vi "classify plclass.vi"(8 "error in":errorcluster, 10 "class cache data in":T1, 11 "Class Ancestry":path[](array[path])) -> (0 "error out":errorcluster, 2 "class cache data out":T1)   [LabVIEW 2013, in "PL_class cache.lvlib"]
uses:
  PL_class cache.lvlib
  cached class information.ctl
  target class metadata.ctl
  class metadata.ctl
  <vilib>/NI/Tag Bus Module Framework/root configuration/Target Types.ctl
  Configuration Editor/Classes/Targets/Targets.lvclass
  <vilib>/NI/Configuration Framework/serializable configuration/NISE_CEF_serializable configuration.lvclass
  Configuration Editor/Classes/Engine Parent/Engine Parent Editor Node.lvclass
  <vilib>/NI/Tag Bus Module Framework/root configuration/TBM configuration.lvclass
  Configuration Editor/Classes/Module editor node/module editor node.lvclass
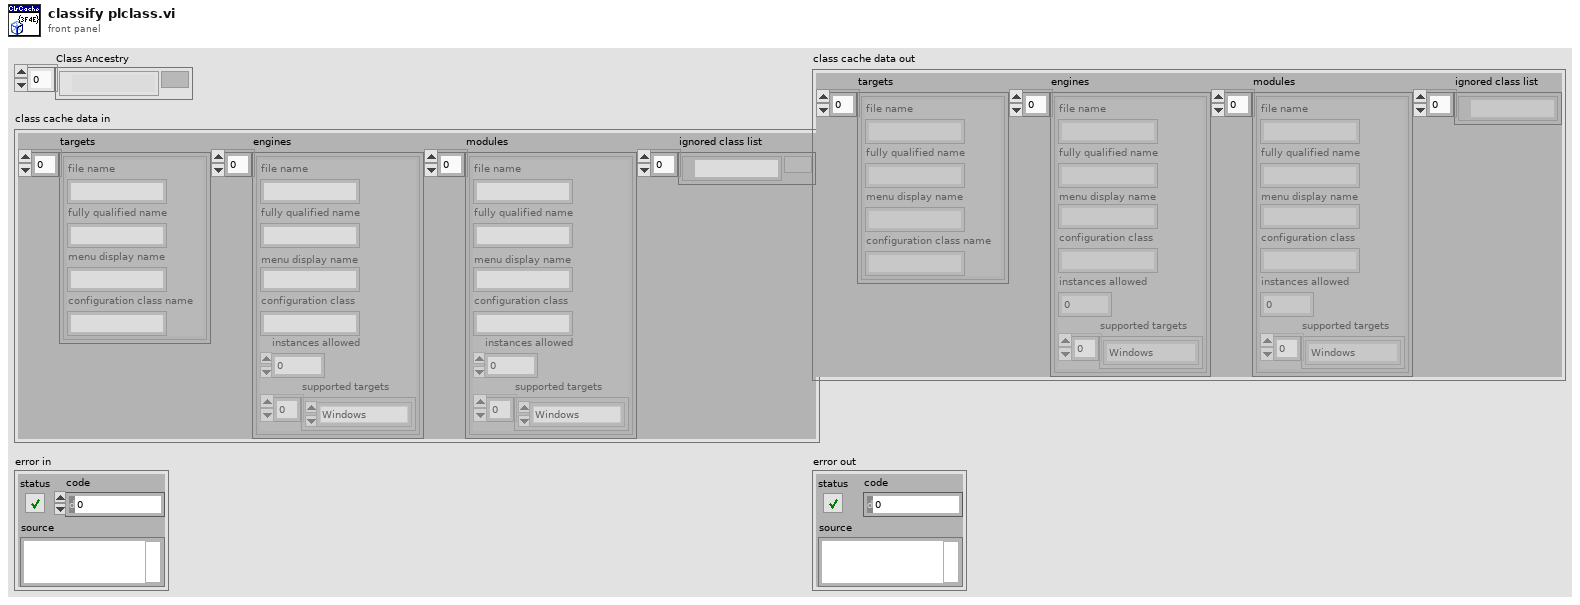
[diagram p1: front panel]
types:
  T1 = typedef "PL_class cache.lvlib/cached class information.ctl" = cluster{"targets":T2[], "engines":T3[], "modules":T3[], "ignored class list":path[]}
  T2 = typedef "PL_class cache.lvlib/target class metadata.ctl" = cluster{"file name":string, "fully qualified name":string, "menu display name":string, "configuration class name":string}
  T3 = typedef "PL_class cache.lvlib/class metadata.ctl" = cluster{"file name":string, "fully qualified name":string, "menu display name":string, "configuration class":string, "instances allowed":i32, "supported targets":T4[]}
  T4 = typedef "TBM configuration.lvclass/Target Types.ctl" = enum16{"Windows", "Mac", "Linux", "Linux RT ARM", "VxWorks", "Pharlap", "Other", "Linux RT x64"}
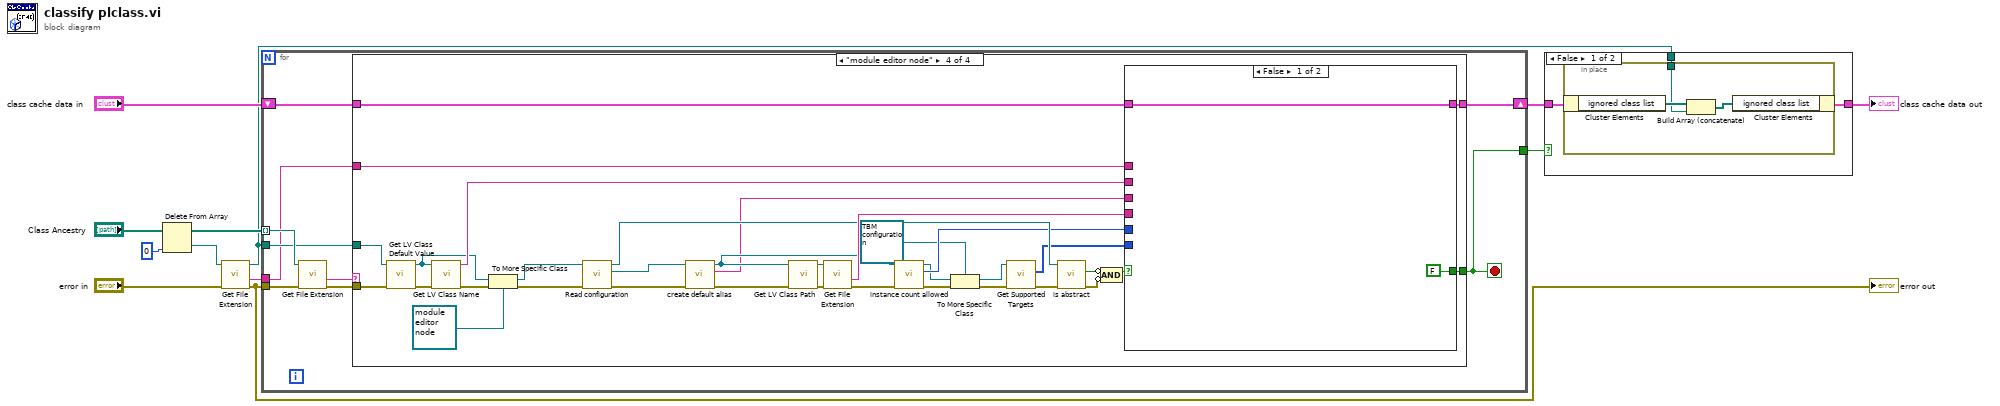
[diagram p0: block diagram]
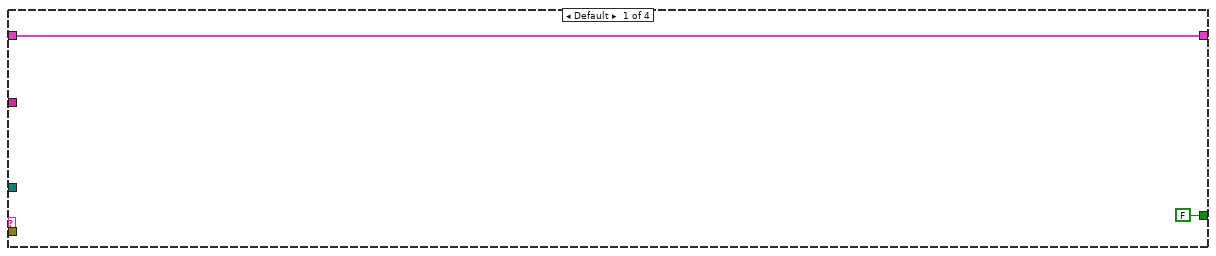
[diagram p3: hidden frame]
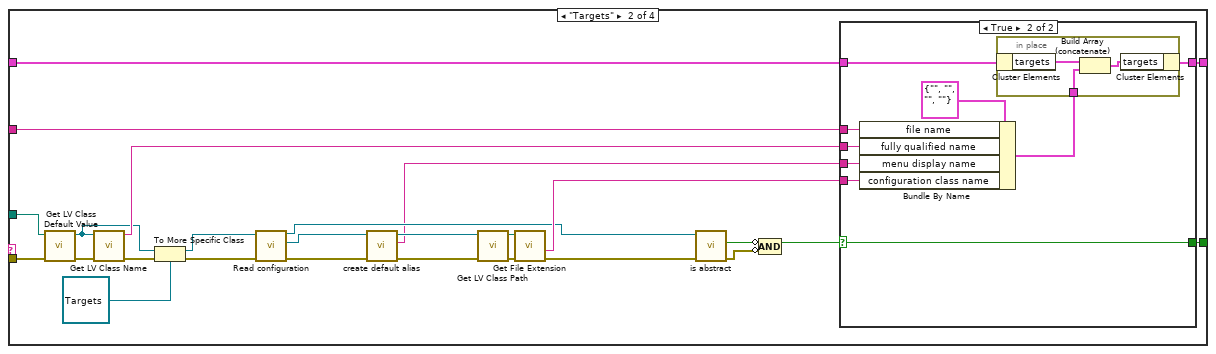
[diagram p4: hidden frame]
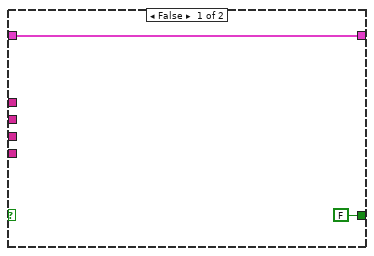
[diagram p5: hidden frame]
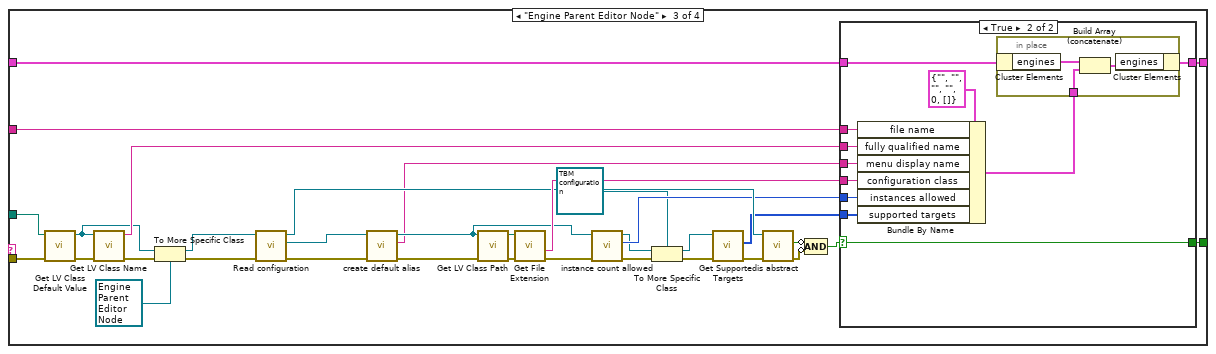
[diagram p6: hidden frame]
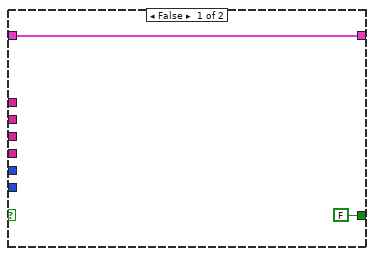
[diagram p7: hidden frame]
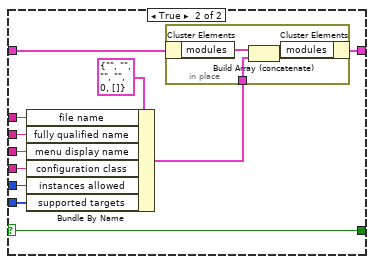
[diagram p8: hidden frame]
diagram:
  n1 = Delete From Array(array="Class Ancestry", index=0) -> (deleted portion=w4:path, array with subset deleted=w11:path[])  [unwired: 1 in]
  n2 = call <vilib>:"Get File Extension.vi"("error in (no error)"="error in", "file"=w4) -> ("error out"=w1:errorcluster, "filename without extension"=w2:string, "dup file"=w3:path)  [unwired: 6 in, 1 out]
  "error out" <- w1
  n3 = for {
    tunnel: w11 -> [w18] mode=indexing
    tunnel: w3 -> [w16]
    shift-right: [w20] -> w6
    shift-left: "class cache data in" -> [w21]
    tunnel: [w14] -> w7
    tunnel: w2 -> [w13]
    tunnel: w1 -> [w15]
    stop <- w14 stop-if-true
    n4 = call <vilib>:"Get File Extension.vi"("error in (no error)"=w15, "file"=w18) -> ("error out"=w19:errorcluster, "filename without extension"=w17:string)  [unwired: 6 in, 2 out]
    n5 = case shown="\"module editor node\"" w17 {
      tunnel: w21 -> [w23 w44 w93 w143]
      tunnel: [w23 w45 w94 w144] -> w20
      tunnel: w19 -> [_ w48 w96 w146]
      tunnel: [FALSE w49 w97 w147] -> w14
      tunnel: w16 -> [_ w47 w95 w145]
      tunnel: w13 -> [_ w43 w92 w142]
      frame Default {
      }
      frame "Targets" {
        n6 = call <vilib>:"Get LV Class Default Value.vi"("error in (no error)"=w48, "class path"=w47) -> ("error out"=w42:errorcluster, "object"=w39:refnum<class>)  [unwired: 8 in]
        n7 = call <vilib>:"Get LV Class Name.vi"("error in (no error)"=w42, "object"=w39) -> ("error out"=w40:errorcluster, "class name"=w41:string)  [unwired: 8 in]
        n8 = To More Specific Class(target class=refnum<class "Targets.lvclass"> refnum ("Targets"), reference=w39, error in=w40) -> (specific class reference=w24:refnum<class "Targets.lvclass">, error out=w25:errorcluster)
        n9 = call-dynamic "Read configuration.vi"("error in"=w25, "NISE_CEF_serializable node in"=w24) -> ("error out"=w37:errorcluster, "configuration"=w28:refnum<class "NISE_CEF_serializable configuration.lvclass">, "NISE_CEF_serializable node out"=w34:refnum<class "Targets.lvclass">)  [unwired: 7 in]
        n10 = call-dynamic "create default alias.vi"("error in"=w37, "configuration in"=w28) -> ("error out"=w29:errorcluster, "default alias"=w26:string, "configuration out"=w27:refnum<class "NISE_CEF_serializable configuration.lvclass">)  [unwired: 7 in]
        n11 = call <vilib>:"Get LV Class Path.vi"("error in (no error)"=w29, "object"=w27) -> ("error out"=w36:errorcluster, "class path"=w38:path)  [unwired: 8 in]
        n12 = call <vilib>:"Get File Extension.vi"("error in (no error)"=w36, "file"=w38) -> ("error out"=w33:errorcluster, "filename without extension"=w35:string)  [unwired: 6 in, 2 out]
        n13 = call-dynamic "is abstract.vi"("error in"=w33, "Targets in"=w34) -> ("error out"=w30:errorcluster, "abstract"=w32:bool)  [unwired: 7 in, 1 out]
        n14 = Compound Arithmetic op=AND(invert w32, invert w30) -> (w31:bool)
        n15 = case shown="True" w31 {
          selector: w31 -> [_ w52]
          tunnel: [FALSE w52] -> w49
          tunnel: [w51 w60] -> w45
          tunnel: w44 -> [w51 w59]
          tunnel: w43 -> [_ w57]
          tunnel: w41 -> [_ w56]
          tunnel: w26 -> [_ w54]
          tunnel: w35 -> [_ w53]
          frame False {
          }
          frame True {
            n16 = Bundle By Name(cluster=T2 {"file name"="", "fully qualified name"="", "menu display name"="", "configuration class name"=""} ("class metadata"), "file name"=w57, "fully qualified name"=w56, "menu display name"=w54, "configuration class name"=w53) -> (w55:T2)
            n17 = in-place {
              in-place-border: w55 -> [w61]
              n18 = in-place-cluster #1(w59) -> ("targets"=w63:T2[])
              n19 = Build Array (concatenate)(w63, w61) -> (w62:T2[])
              n20 = in-place-cluster #1("targets"=w62) -> (w60:T1)
            }
          }
        }
      }
      frame "Engine Parent Editor Node" {
        n21 = call <vilib>:"Get LV Class Default Value.vi"("error in (no error)"=w96, "class path"=w95) -> ("error out"=w91:errorcluster, "object"=w88:refnum<class>)  [unwired: 8 in]
        n22 = call <vilib>:"Get LV Class Name.vi"("error in (no error)"=w91, "object"=w88) -> ("error out"=w89:errorcluster, "class name"=w90:string)  [unwired: 8 in]
        n23 = To More Specific Class(target class=refnum<class "Engine Parent Editor Node.lvclass"> refnum ("Engine Parent.lvclass"), reference=w88, error in=w89) -> (specific class reference=w64:refnum<class "Engine Parent Editor Node.lvclass">, error out=w65:errorcluster)
        n24 = call-dynamic "Read configuration.vi"("error in"=w65, "NISE_CEF_serializable node in"=w64) -> ("error out"=w86:errorcluster, "configuration"=w68:refnum<class "NISE_CEF_serializable configuration.lvclass">, "NISE_CEF_serializable node out"=w83:refnum<class "Engine Parent Editor Node.lvclass">)  [unwired: 7 in]
        n25 = call-dynamic "create default alias.vi"("error in"=w86, "configuration in"=w68) -> ("error out"=w69:errorcluster, "default alias"=w66:string, "configuration out"=w67:refnum<class "NISE_CEF_serializable configuration.lvclass">)  [unwired: 7 in]
        n26 = call <vilib>:"Get LV Class Path.vi"("error in (no error)"=w69, "object"=w67) -> ("error out"=w85:errorcluster, "class path"=w87:path)  [unwired: 8 in]
        n27 = call <vilib>:"Get File Extension.vi"("error in (no error)"=w85, "file"=w87) -> ("error out"=w82:errorcluster, "filename without extension"=w84:string)  [unwired: 6 in, 2 out]
        n28 = call-dynamic "instance count allowed.vi"("error in"=w82, "configuration in"=w67) -> ("error out"=w79:errorcluster, "instances allowed"=w76:i32, "configuration out"=w71:refnum<class "NISE_CEF_serializable configuration.lvclass">)  [unwired: 7 in]
        n29 = To More Specific Class(target class=refnum<class "TBM configuration.lvclass"> refnum ("configuration in"), reference=w71, error in=w79) -> (specific class reference=w70:refnum<class "TBM configuration.lvclass">, error out=w73:errorcluster)
        n30 = call-dynamic "Get Supported Targets.vi"("error in"=w73, "configuration in"=w70) -> ("error out"=w78:errorcluster, "supported targets"=w77:T4[])  [unwired: 7 in, 1 out]
        n31 = call-dynamic "is abstract.vi"("error in"=w78, "Engine Parent Editor Node in"=w83) -> ("error out"=w74:errorcluster, "abstract"=w81:bool)  [unwired: 7 in, 1 out]
        n32 = Compound Arithmetic op=AND(invert w81, invert w74) -> (w75:bool)
        n33 = case shown="True" w75 {
          selector: w75 -> [_ w103]
          tunnel: [FALSE w103] -> w97
          tunnel: [w99 w110] -> w94
          tunnel: w93 -> [w99 w109]
          tunnel: w92 -> [_ w108]
          tunnel: w90 -> [_ w107]
          tunnel: w66 -> [_ w105]
          tunnel: w84 -> [_ w104]
          tunnel: w77 -> [_ w101]
          tunnel: w76 -> [_ w100]
          frame False {
          }
          frame True {
            n34 = Bundle By Name(cluster=T3 {"file name"="", "fully qualified name"="", "menu display name"="", "configuration class"="", "instances allowed"=0, "supported targets"=[]} ("class metadata"), "file name"=w108, "fully qualified name"=w107, "menu display name"=w105, "configuration class"=w104, "instances allowed"=w100, "supported targets"=w101) -> (w106:T3)
            n35 = in-place {
              in-place-border: w106 -> [w111]
              n36 = in-place-cluster #2(w109) -> ("engines"=w113:T3[])
              n37 = Build Array (concatenate)(w113, w111) -> (w112:T3[])
              n38 = in-place-cluster #2("engines"=w112) -> (w110:T1)
            }
          }
        }
      }
      frame "module editor node" {
        n39 = call <vilib>:"Get LV Class Default Value.vi"("error in (no error)"=w146, "class path"=w145) -> ("error out"=w141:errorcluster, "object"=w138:refnum<class>)  [unwired: 8 in]
        n40 = call <vilib>:"Get LV Class Name.vi"("error in (no error)"=w141, "object"=w138) -> ("error out"=w139:errorcluster, "class name"=w140:string)  [unwired: 8 in]
        n41 = To More Specific Class(target class=refnum<class "module editor node.lvclass"> refnum ("Component Parent.lvclass"), reference=w138, error in=w139) -> (specific class reference=w114:refnum<class "module editor node.lvclass">, error out=w115:errorcluster)
        n42 = call-dynamic "Read configuration.vi"("error in"=w115, "NISE_CEF_serializable node in"=w114) -> ("error out"=w136:errorcluster, "configuration"=w118:refnum<class "NISE_CEF_serializable configuration.lvclass">, "NISE_CEF_serializable node out"=w133:refnum<class "module editor node.lvclass">)  [unwired: 7 in]
        n43 = call-dynamic "create default alias.vi"("error in"=w136, "configuration in"=w118) -> ("error out"=w119:errorcluster, "default alias"=w116:string, "configuration out"=w117:refnum<class "NISE_CEF_serializable configuration.lvclass">)  [unwired: 7 in]
        n44 = call <vilib>:"Get LV Class Path.vi"("error in (no error)"=w119, "object"=w117) -> ("error out"=w135:errorcluster, "class path"=w137:path)  [unwired: 8 in]
        n45 = call <vilib>:"Get File Extension.vi"("error in (no error)"=w135, "file"=w137) -> ("error out"=w132:errorcluster, "filename without extension"=w134:string)  [unwired: 6 in, 2 out]
        n46 = call-dynamic "instance count allowed.vi"("error in"=w132, "configuration in"=w117) -> ("error out"=w130:errorcluster, "instances allowed"=w127:i32, "configuration out"=w122:refnum<class "NISE_CEF_serializable configuration.lvclass">)  [unwired: 7 in]
        n47 = To More Specific Class(target class=refnum<class "TBM configuration.lvclass"> refnum ("configuration in"), reference=w122, error in=w130) -> (specific class reference=w120:refnum<class "TBM configuration.lvclass">, error out=w123:errorcluster)
        n48 = call-dynamic "Get Supported Targets.vi"("error in"=w123, "configuration in"=w120) -> ("error out"=w129:errorcluster, "supported targets"=w128:T4[])  [unwired: 7 in, 1 out]
        n49 = call-dynamic "is abstract.vi"("error in"=w129, "module editor node in"=w133) -> ("error out"=w124:errorcluster, "abstract"=w131:bool)  [unwired: 7 in, 1 out]
        n50 = Compound Arithmetic op=AND(invert w131, invert w124) -> (w125:bool)
        n51 = case shown="False" w125 {
          selector: w125 -> [_ w153]
          tunnel: [FALSE w153] -> w147
          tunnel: [w149 w160] -> w144
          tunnel: w143 -> [w149 w159]
          tunnel: w142 -> [_ w158]
          tunnel: w140 -> [_ w157]
          tunnel: w116 -> [_ w155]
          tunnel: w134 -> [_ w154]
          tunnel: w128 -> [_ w151]
          tunnel: w127 -> [_ w150]
          frame False {
          }
          frame True {
            n52 = Bundle By Name(cluster=T3 {"file name"="", "fully qualified name"="", "menu display name"="", "configuration class"="", "instances allowed"=0, "supported targets"=[]} ("class metadata"), "file name"=w158, "fully qualified name"=w157, "menu display name"=w155, "configuration class"=w154, "instances allowed"=w150, "supported targets"=w151) -> (w156:T3)
            n53 = in-place {
              in-place-border: w156 -> [w161]
              n54 = in-place-cluster #3(w159) -> ("modules"=w163:T3[])
              n55 = Build Array (concatenate)(w163, w161) -> (w162:T3[])
              n56 = in-place-cluster #3("modules"=w162) -> (w160:T1)
            }
          }
        }
      }
    }
  }
  n57 = case shown="False" w7 {
    tunnel: w6 -> [w166 w170]
    tunnel: [w165 w170] -> w5
    tunnel: w3 -> [w164 _]
    frame False {
      n58 = in-place {
        in-place-border: w164 -> [w167]
        n59 = in-place-cluster #4(w166) -> ("ignored class list"=w169:path[])
        n60 = Build Array (concatenate)(w169, w167) -> (w168:path[])
        n61 = in-place-cluster #4("ignored class list"=w168) -> (w165:T1)
      }
    }
    frame True {
      # "success"
    }
  }
  "class cache data out" <- w5
